vi "Mecanum Robot Body Model.vi"(11 "ccw torques":dbl[](array[numeric])=[1.0, -1.0, -1.0, 1.0]) -> (0 "theta 2":dbl, 1 "x,y (inertial)":dbl[](array[numeric])=[0.0, 200.0], 2 "theta'":dbl, 3 "x',y' (inertial)":dbl[](array[numeric])=[0.0, 200.0], 4 "ccw wheel angles":dbl[](array[numeric])=[200.0, -200.0, -200.0, 200.0], 5 "ccw wheel angular velocities":dbl[](array[numeric])=[40.0, -40.0, -40.0, 40.0])   [LabVIEW 2017]
uses:
  <vilib>/Simulation/Implementation/Shared/SIMSCR Execution Mode.ctl
  <vilib>/Simulation/Scripting/Companion Diagram/SimConfigNode/SimParams.ctl
  <vilib>/Simulation/Scripting/Companion Diagram/SimConfigNode/_simSolvers.ctl
  <vilib>/Simulation/Param Hierarchy/Typedefs/SIMPH Param Control Actions.ctl
  <vilib>/Analysis/Matrix/Datatypes/RealMatrix.ctl
  <vilib>/Simulation/Implementation/Shared/SIM limit type.ctl
  <vilib>/Simulation/Implementation/Shared/NILVSim_ParamChanged.vi
  <vilib>/Simulation/Implementation/Shared/NILVSIM_BeginStep.vi
  <vilib>/Analysis/baseanly.llb/A x Vector.vi
  <vilib>/Simulation/ContinuousLinear/Implementation/NILVSim Integrator new.llb/SIM Integrator distributor (scalar).vi
  <vilib>/Simulation/ContinuousLinear/Implementation/NILVSim Integrator new.llb/SIM Integrator collector (scalar).vi
  <vilib>/Analysis/coordinate.llb/2D Cartesian Coordinate Rotation (Scalar).vi
  <vilib>/Simulation/ContinuousLinear/Implementation/NILVSim Integrator new.llb/SIM Integrator Distributor (vector).vi
  <vilib>/Simulation/ContinuousLinear/Implementation/NILVSim Integrator new.llb/SIM Integrator Collector (vector).vi
  <vilib>/Simulation/Implementation/Shared/NILVSim_Manager.vi
  <vilib>/Utility/error.llb/Clear Errors.vi
  <vilib>/Simulation/Implementation/Shared/NILVSim_FinalizeModel.vi
  <vilib>/Simulation/Implementation/Shared/SIM Unbundle Sim Info.vi
  <vilib>/Simulation/Implementation/Shared/SIMSH Read Queue.vi
  Robot Parameters/Robot Parameters.vi
  <vilib>/Simulation/Implementation/Shared/NILVSim_Initialize.vi
  <vilib>/Simulation/Utility/Implementation/NILVSim Get Time and IsAcceptedStep.vi
  <vilib>/Simulation/Implementation/Shared/NILVSim_GetModelError.vi
  <vilib>/Simulation/Implementation/Shared/SIM SimErrorHandler.vi
  <vilib>/Simulation/Implementation/Shared/SIM Bundle Sim Info.vi
  <vilib>/Simulation/Scripting/Companion Diagram/SimConfigNode/SimDog.xnode
  <vilib>/Analysis/NI_AALPro.lvlib
  <vilib>/Analysis/NI_AALBase.lvlib
  <vilib>/Analysis/Matrix/NI_Matrix.lvlib
  <vilib>/Simulation/Implementation/XNodeFramework/SimXNode/SimX.xnode
  <vilib>/Simulation/ContinuousLinear/Implementation/NILVSim Integrator new.llb/SIM Integrator (scalar).vi
  <vilib>/Simulation/ContinuousLinear/Implementation/NILVSim Integrator new.llb/SIM Integrator (vector).vi
  <vilib>/Simulation/Implementation/Shared/NI_SIM_Implementation.lvlib
panel:
  # "Motor Torques, in clockwise order from top left"
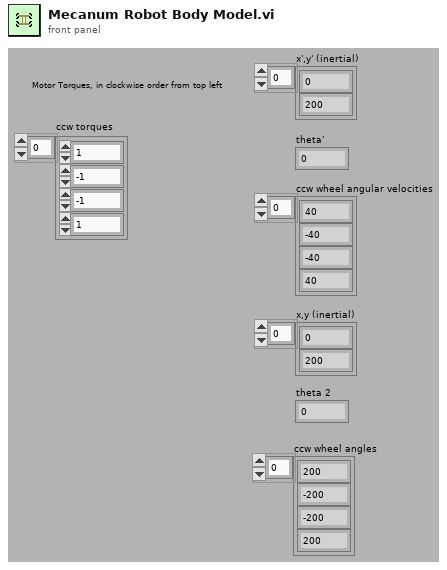
[diagram p1: front panel]
types:
  T1 = typedef "NI_Matrix.lvlib/RealMatrix.ctl" = dbl[][]
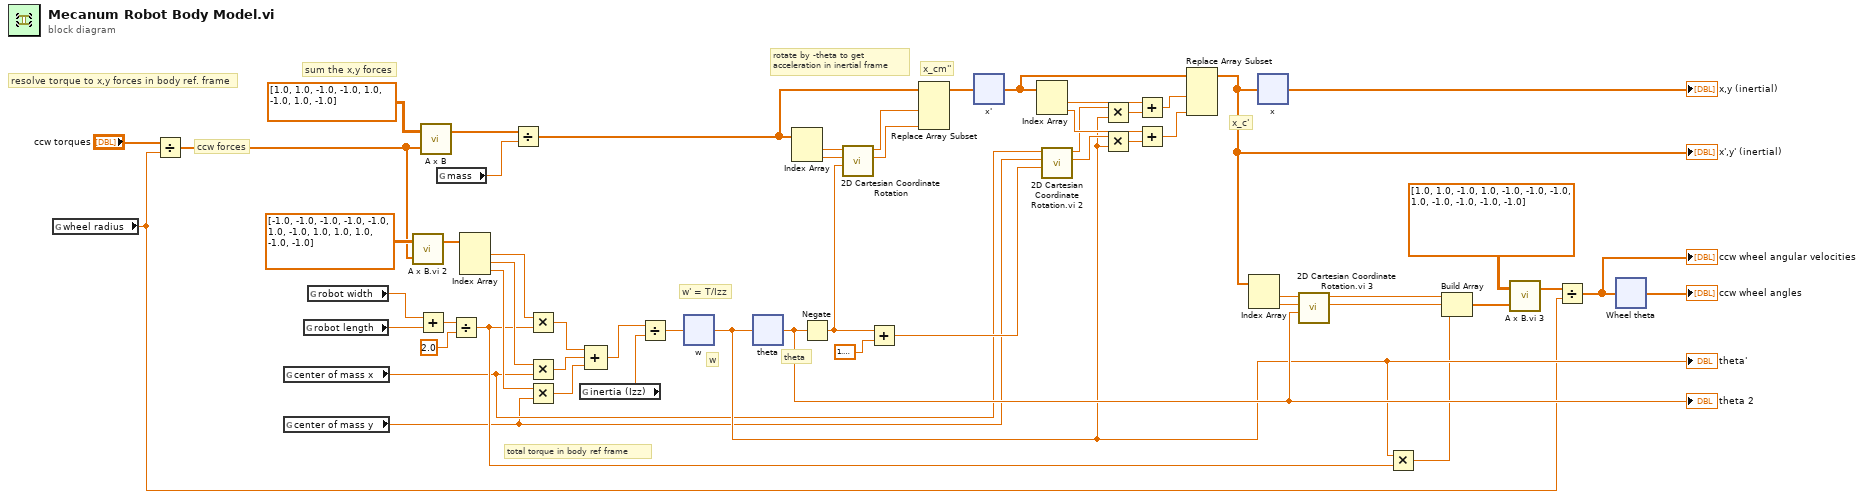
[diagram p0: block diagram]
diagram:
  # "ccw forces"
  # "sum the x,y forces"
  # "x_c'"
  # "x_cm''"
  # "rotate by -theta to get\nacceleration in inertial frame"
  # "theta"
  # "w"
  # "w' = T/Izz"
  # "total torque in body ref frame"
  # "resolve torque to x,y forces in body ref. frame"
  n1 = global read "Robot Parameters.vi" "wheel radius"() -> (w7:dbl)
  n2 = Divide ("Divide 3")(x="ccw torques", y=w7) -> (x/y=w43:dbl[])
  n3 = global read "Robot Parameters.vi 4" "center of mass x"() -> (w4:dbl)
  n4 = global read "Robot Parameters.vi 5" "center of mass y"() -> (w3:dbl)
  n5 = global read "Robot Parameters.vi 3" "robot length"() -> (w6:dbl)
  n6 = global read "Robot Parameters.vi 2" "robot width"() -> (w5:dbl)
  n7 = call-poly "A x B.vi 2"("Vector"=w43, "A"=T1 [[-1.0, -1.0, -1.0, -1.0], [-1.0, 1.0, -1.0, 1.0], [1.0, 1.0, -1.0, -1.0]]) -> ("A x Vector"=w42:dbl[])  [unwired: 1 out]
  n8 = Add ("Add 4")(x=w5, y=w6) -> (x+y=w18:dbl)
  n9 = call-poly <vilib>:"A x B.vi"("Vector"=w43, "A"=T1 [[1.0, 1.0, -1.0, -1.0], [1.0, -1.0, 1.0, -1.0]] ("A 2")) -> ("A x Vector"=w47:dbl[])  [unwired: 1 out]
  n10 = global read "Robot Parameters.vi 7" "mass"() -> (w1:dbl)
  n11 = Divide ("Divide 4")(x=w18, y=2.0) -> (x/y=w15:dbl)
  n12 = Index Array ("Index Array 2")(array=w42) -> (element #1=w41:dbl, element #2=w40:dbl, element #3=w39:dbl)  [unwired: 3 in]
  n13 = Divide ("Divide 2")(x=w47, y=w1) -> (x/y=w51:dbl[])
  n14 = Multiply(x=w41, y=w15) -> (x*y=w38:dbl)
  n15 = Multiply ("Multiply 2")(x=w40, y=w4) -> (x*y=w37:dbl)
  n16 = Multiply ("Multiply 3")(x=w39, y=w3) -> (x*y=w36:dbl)
  n17 = global read "Robot Parameters.vi 6" "inertia (Izz)"() -> (w2:dbl)
  n18 = Compound Arithmetic op=ADD(w38, w37, w36) -> (w35:dbl)
  n19 = Divide(x=w35, y=w2) -> (x/y=w56:dbl)
  n20 = xnode "w"("input"=w56) -> ("output"=w16:dbl)  [unwired: 9 in, 2 out]
  "theta'" <- w16
  n21 = xnode "theta"("input"=w16) -> ("output"=w19:dbl)  [unwired: 9 in, 2 out]
  "theta 2" <- w19
  n22 = Index Array(array=w51) -> (element #1=w55:dbl, element #2=w54:dbl)  [unwired: 2 in]
  n23 = Negate(x=w19) -> (-x=w33:dbl)
  n24 = call-poly <vilib>:"2D Cartesian Coordinate Rotation.vi"("theta"=w33, "y"=w54, "x"=w55) -> ("y out"=w52:dbl, "x out"=w53:dbl)  [unwired: 6 in, 1 out]
  n25 = Add ("Add 2")(x=w33, y=1.5707963267948966 ("Constant")) -> (x+y=w31:dbl)
  n26 = Replace Array Subset(array=w51, new element #1=w53, new element #2=w52) -> (w50:dbl[])  [unwired: 2 in]
  n27 = xnode "x'"("input"=w50) -> ("output"=w34:dbl[])  [unwired: 9 in, 2 out]
  n28 = Index Array ("Index Array 3")(array=w34) -> (element #1=w30:dbl, element #2=w29:dbl)  [unwired: 2 in]
  n29 = call-poly "2D Cartesian Coordinate Rotation.vi 2"("theta"=w31, "y"=w3, "x"=w4) -> ("y out"=w26:dbl, "x out"=w28:dbl)  [unwired: 6 in, 1 out]
  n30 = Multiply ("Multiply 4")(x=w28, y=w16) -> (x*y=w27:dbl)
  n31 = Multiply ("Multiply 5")(x=w26, y=w16) -> (x*y=w25:dbl)
  n32 = Add(x=w30, y=w27) -> (x+y=w24:dbl)
  n33 = Add ("Add 3")(x=w29, y=w25) -> (x+y=w23:dbl)
  n34 = Replace Array Subset ("Replace Array Subset 2")(array=w34, new element #1=w24, new element #2=w23) -> (w20:dbl[])  [unwired: 2 in]
  "x',y' (inertial)" <- w20
  n35 = Index Array ("Index Array 4")(array=w20) -> (element #1=w22:dbl, element #2=w21:dbl)  [unwired: 2 in]
  n36 = xnode "x"("input"=w20) -> ("output"=→"x,y (inertial)":dbl[])  [unwired: 9 in, 2 out]
  n37 = call-poly "2D Cartesian Coordinate Rotation.vi 3"("theta"=w19, "y"=w21, "x"=w22) -> ("y out"=w12:dbl, "x out"=w13:dbl)  [unwired: 7 out]
  n38 = Multiply ("Multiply 6")(x=w16, y=w15) -> (x*y=w14:dbl)
  n39 = Build Array(w13, w12, w14) -> (w11:dbl[])
  n40 = call-poly "A x B.vi 3"("Vector"=w11, "A"=dbl[][] [[1.0, 1.0, -1.0], [1.0, -1.0, -1.0], [-1.0, 1.0, -1.0], [-1.0, -1.0, -1.0]] ("Constant 2")) -> ("A x Vector"=w9:dbl[])  [unwired: 1 out]
  n41 = Divide ("Divide 5")(x=w9, y=w7) -> (x/y=w8:dbl[])
  "ccw wheel angular velocities" <- w8
  n42 = xnode "Wheel theta"("input"=w8) -> ("output"=→"ccw wheel angles":dbl[])  [unwired: 9 in, 2 out]
